vi "P.vi"(8 "change time":dbl, 9 "P gain":dbl, 11 "error":dbl) -> (1 "output":dbl)   [LabVIEW 2009]
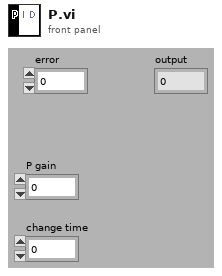
[diagram p1: front panel]
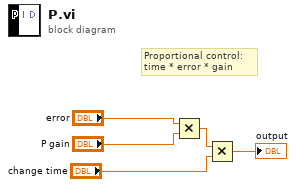
[diagram p0: block diagram]
diagram:
  # "Proportional control:\ntime * error * gain"
  n1 = Multiply(x="error", y="P gain") -> (x*y=w4:dbl)
  n2 = Multiply(x=w4, y="change time") -> (x*y=→"output":dbl)
